vi "closeDump.vi"(1 "relay session in":T1={"VISA resource out"="COM12", "error out"={"status"=FALSE, "code"=0, "source"=""}}) -> (0 "relay session out":T1={"VISA resource out"="COM12", "error out"={"status"=FALSE, "code"=0, "source"=""}})   [LabVIEW 2010]
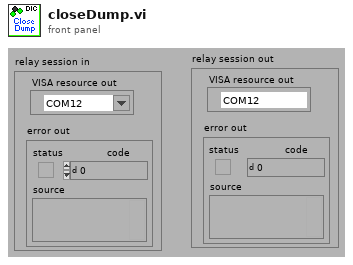
[diagram p1: front panel]
types:
  T1 = cluster{"VISA resource out":refnum<visa-resource-name>, "error out":errorcluster}
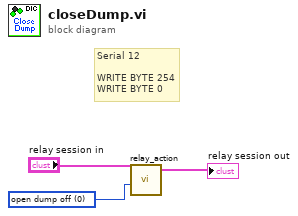
[diagram p0: block diagram]
diagram:
  w1 = u8 0 items=["open dump on"=8, "pump acid on"=9, "air flush on"=10, "stop gas flow on"=11, "open dump off"=0, "pump acid off"=1, "air flush off"=2, "stop gas flow off"=3, "OpenAll"=30, "CloseAll"=29] ("Action")
  # "Serial 12\n\nWRITE BYTE 254\nWRITE BYTE 0"
  n1 = call "relay_action.vi"("relay session in"="relay session in", "Action"=w1) -> ("relay session out"=→"relay session out":T1)  [unwired: 6 in]
